vi "subvi_read_angle.vi"(11 "file (use dialog)":path) -> (3 "Current Angles":cluster{"Analyser 1":i32, "Analyser 2":i32})   [LabVIEW 2014]
doc: "Reads the first two numbers from a txt file seperated by a comma on a newline and outputs these two numbers as a cluster."
uses:
  <vilib>/Utility/file.llb/Read From Spreadsheet File (I64).vi
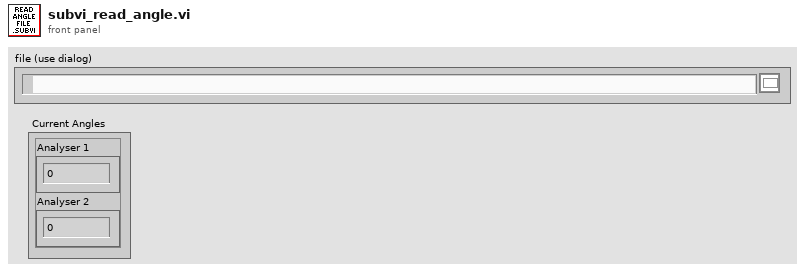
[diagram p1: front panel]
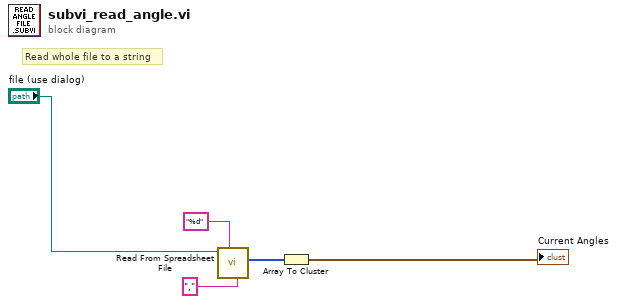
[diagram p0: block diagram]
diagram:
  # "Read whole file to a string"
  n1 = call-poly <vilib>:"Read From Spreadsheet File.vi"("delimiter (\\t)"="," ("delimiter (\\t)"), "format (%d)"="%d", "file path (dialog if empty)"="file (use dialog)") -> ("first row"=w2:i64[])  [unwired: 4 in, 4 out]
  n2 = Array To Cluster(array=w2) -> (cluster=→"Current Angles":cluster{"first row[0]":i64, "first row[1]":i64})
